vi "Mod_OFDM_Config_Data_Source.vi"(0 "Configuration in":variant=variant("Attribute Names"=variant(cluster{"Data Source Pool":string, "Modulator Source Pool":string, "OFDM SYMBOL POOL":string, "Symbol Table":string, "Sub Carrier Selection":string, "OFDM Frame":string, "FRAME Table":string, "Pulse Shaping":string} {"Data Source Pool"="Data Source ", "Modulator Source Pool"="Modulator Source Pool ", "OFDM SYMBOL POOL"="OFDM SYMBOL POOL", "Symbol Table"="Symbol Table", "Sub Carrier Selection"="Sub Carrier Selection", "OFDM Frame"="OFDM Frame", "FRAME Table"="FRAME Table", "Pulse Shaping"="Pulse Shaping"}), "Data Source "=variant(cluster{"mode (PN)":enum16{"PN", "pattern", "user"}, "PN sequence order (9)":i32, "Invert Output Bits":enum16{"No", "Yes"}, "Register Initial State":u32, "User base bit pattern":i8[], "base bit pattern (00001111)":enum16{"0", "1", "01", "0011", "00001111"}, "Reset to Initial State":enum16{"Every OFDM Frame", "Every OFDM Symbol", "Every Sub Carrier"}}[] [{"mode (PN)"=enum."PN", "PN sequence order (9)"=9, "Invert Output Bits"=enum."No", "Register Initial State"=3602873842, "User base bit pattern"=[], "base bit pattern (00001111)"=enum."00001111", "Reset to Initial State"=enum."Every OFDM Frame"}, {"mode (PN)"=enum."PN", "PN sequence order (9)"=9, "Invert Output Bits"=enum."No", "Register Initial State"=3602873842, "User base bit pattern"=[], "base bit pattern (00001111)"=enum."00001111", "Reset to Initial State"=enum."Every OFDM Frame"}, {"mode (PN)"=enum."PN", "PN sequence order (9)"=9, "Invert Output Bits"=enum."No", "Register Initial State"=3602873842, "User base bit pattern"=[], "base bit pattern (00001111)"=enum."00001111", "Reset to Initial State"=enum."Every OFDM Frame"}, {"mode (PN)"=enum."PN", "PN sequence order (9)"=9, "Invert Output Bits"=enum."No", "Register Initial State"=3602873842, "User base bit pattern"=[], "base bit pattern (00001111)"=enum."00001111", "Reset to Initial State"=enum."Every OFDM Frame"}]), "FRAME Table"=variant(string[][] [["No_Name", "  1", "  1"], ["No_Name", "  1", "  2"]]), "Modulator Source Pool "=variant(cluster{"M-QAM":enum16{"4", "16", "64", "256"}, "M-PSK":enum16{"2", "4", "8", "16", "32", "64", "128", "256"}, "Type of Modulation":enum16{"PSK", "QAM"}, "PSK":cluster{"differential PSK":enum16{"disable", "enable"}, "PSK type":enum16{"normal", "shifted", "offset"}}}[] [{"M-QAM"=enum."4", "M-PSK"=enum."2", "Type of Modulation"=enum."PSK", "PSK"={"differential PSK"=enum."disable", "PSK type"=enum."normal"}}, {"M-QAM"=enum."4", "M-PSK"=enum."2", "Type of Modulation"=enum."PSK", "PSK"={"differential PSK"=enum."disable", "PSK type"=enum."normal"}}, {"M-QAM"=enum."4", "M-PSK"=enum."2", "Type of Modulation"=enum."PSK", "PSK"={"differential PSK"=enum."disable", "PSK type"=enum."normal"}}, {"M-QAM"=enum."4", "M-PSK"=enum."2", "Type of Modulation"=enum."PSK", "PSK"={"differential PSK"=enum."disable", "PSK type"=enum."normal"}}]), "No_Name"=variant(cluster{"Sub Carrier Selection":cluster{"Sub Carrier":bool, "Data Source":u16, "Modulator":u16}[], "OFDM Parameters":cluster{"# of Sub Carrier":i32, "Length Of Cylic Prefix":i32}} {"Sub Carrier Selection"=[{"Sub Carrier"=TRUE, "Data Source"=0, "Modulator"=0}, {"Sub Carrier"=TRUE, "Data Source"=0, "Modulator"=0}, {"Sub Carrier"=TRUE, "Data Source"=0, "Modulator"=0}, {"Sub Carrier"=TRUE, "Data Source"=0, "Modulator"=0}, {"Sub Carrier"=TRUE, "Data Source"=0, "Modulator"=0}, {"Sub Carrier"=TRUE, "Data Source"=0, "Modulator"=0}, {"Sub Carrier"=TRUE, "Data Source"=0, "Modulator"=0}, {"Sub Carrier"=TRUE, "Data Source"=0, "Modulator"=0}, {"Sub Carrier"=TRUE, "Data Source"=0, "Modulator"=0}, {"Sub Carrier"=TRUE, "Data Source"=0, "Modulator"=0}, {"Sub Carrier"=TRUE, "Data Source"=0, "Modulator"=0}, {"Sub Carrier"=TRUE, "Data Source"=0, "Modulator"=0}, {"Sub Carrier"=TRUE, "Data Source"=0, "Modulator"=0}, {"Sub Carrier"=TRUE, "Data Source"=0, "Modulator"=0}, {"Sub Carrier"=TRUE, "Data Source"=0, "Modulator"=0}, {"Sub Carrier"=TRUE, "Data Source"=0, "Modulator"=0}, {"Sub Carrier"=TRUE, "Data Source"=0, "Modulator"=0}, {"Sub Carrier"=TRUE, "Data Source"=0, "Modulator"=0}, {"Sub Carrier"=TRUE, "Data Source"=0, "Modulator"=0}, {"Sub Carrier"=TRUE, "Data Source"=0, "Modulator"=0}, {"Sub Carrier"=TRUE, "Data Source"=0, "Modulator"=0}, {"Sub Carrier"=TRUE, "Data Source"=0, "Modulator"=0}, {"Sub Carrier"=TRUE, "Data Source"=0, "Modulator"=0}, {"Sub Carrier"=TRUE, "Data Source"=0, "Modulator"=0}, {"Sub Carrier"=TRUE, "Data Source"=0, "Modulator"=0}, {"Sub Carrier"=TRUE, "Data Source"=0, "Modulator"=0}, {"Sub Carrier"=TRUE, "Data Source"=0, "Modulator"=0}, {"Sub Carrier"=TRUE, "Data Source"=0, "Modulator"=0}, {"Sub Carrier"=TRUE, "Data Source"=0, "Modulator"=0}, {"Sub Carrier"=TRUE, "Data Source"=0, "Modulator"=0}, {"Sub Carrier"=TRUE, "Data Source"=0, "Modulator"=0}, {"Sub Carrier"=TRUE, "Data Source"=0, "Modulator"=0}, {"Sub Carrier"=TRUE, "Data Source"=0, "Modulator"=0}, {"Sub Carrier"=TRUE, "Data Source"=0, "Modulator"=0}, {"Sub Carrier"=TRUE, "Data Source"=0, "Modulator"=0}, {"Sub Carrier"=TRUE, "Data Source"=0, "Modulator"=0}, {"Sub Carrier"=TRUE, "Data Source"=0, "Modulator"=0}, {"Sub Carrier"=TRUE, "Data Source"=0, "Modulator"=0}, {"Sub Carrier"=TRUE, "Data Source"=0, "Modulator"=0}, {"Sub Carrier"=TRUE, "Data Source"=0, "Modulator"=0}, {"Sub Carrier"=TRUE, "Data Source"=0, "Modulator"=0}, {"Sub Carrier"=TRUE, "Data Source"=0, "Modulator"=0}, {"Sub Carrier"=TRUE, "Data Source"=0, "Modulator"=0}, {"Sub Carrier"=TRUE, "Data Source"=0, "Modulator"=0}, {"Sub Carrier"=TRUE, "Data Source"=0, "Modulator"=0}, {"Sub Carrier"=TRUE, "Data Source"=0, "Modulator"=0}, {"Sub Carrier"=TRUE, "Data Source"=0, "Modulator"=0}, {"Sub Carrier"=TRUE, "Data Source"=0, "Modulator"=0}, {"Sub Carrier"=TRUE, "Data Source"=0, "Modulator"=0}, {"Sub Carrier"=TRUE, "Data Source"=0, "Modulator"=0}, {"Sub Carrier"=TRUE, "Data Source"=0, "Modulator"=0}, {"Sub Carrier"=TRUE, "Data Source"=0, "Modulator"=0}, {"Sub Carrier"=TRUE, "Data Source"=0, "Modulator"=0}, {"Sub Carrier"=TRUE, "Data Source"=0, "Modulator"=0}, {"Sub Carrier"=TRUE, "Data Source"=0, "Modulator"=0}, {"Sub Carrier"=TRUE, "Data Source"=0, "Modulator"=0}, {"Sub Carrier"=TRUE, "Data Source"=0, "Modulator"=0}, {"Sub Carrier"=TRUE, "Data Source"=0, "Modulator"=0}, {"Sub Carrier"=TRUE, "Data Source"=0, "Modulator"=0}, {"Sub Carrier"=TRUE, "Data Source"=0, "Modulator"=0}, {"Sub Carrier"=TRUE, "Data Source"=0, "Modulator"=0}, {"Sub Carrier"=TRUE, "Data Source"=0, "Modulator"=0}, {"Sub Carrier"=TRUE, "Data Source"=0, "Modulator"=0}, {"Sub Carrier"=TRUE, "Data Source"=0, "Modulator"=0}], "OFDM Parameters"={"# of Sub Carrier"=64, "Length Of Cylic Prefix"=16}}), "OFDM Frame"=variant(cluster{"Symbol Name":string, "# of Symbols":i32}[] [{"Symbol Name"="No_Name", "# of Symbols"=1}, {"Symbol Name"="No_Name", "# of Symbols"=1}]), "OFDM SYMBOL POOL"=variant(string[] ["No_Name"]), "Pulse Shaping"=variant(cluster{"System Filter":cluster{"TX Filter":enum16{"none", "Raised Cosine", "Root Raised Cos"}, "Alpha":dbl, "filter length":i32}, "Modulation system parameters":cluster{"samples per symbol (16)":u32}, "symbol rate (Hz)":dbl} {"System Filter"={"TX Filter"=enum."Root Raised Cos", "Alpha"=0.5, "filter length"=8}, "Modulation system parameters"={"samples per symbol (16)"=16}, "symbol rate (Hz)"=100000.0}), "Sub Carrier Selection"=variant(cluster{"Sub Carrier Selection":cluster{"Sub Carrier":bool, "Data Source":u16, "Modulator":u16}[], "OFDM Parameters":cluster{"# of Sub Carrier":i32, "Length Of Cylic Prefix":i32}} {"Sub Carrier Selection"=array[10000 elements], "OFDM Parameters"={"# of Sub Carrier"=64, "Length Of Cylic Prefix"=16}}), "Symbol Table"=variant(string[][] [["-32", " ON", "0", "0"], ["-31", " ON", "0", "0"], ["-30", " ON", "0", "0"], ["-29", " ON", "0", "0"], ["-28", " ON", "0", "0"], ["-27", " ON", "0", "0"], ["-26", " ON", "0", "0"], ["-25", " ON", "0", "0"], ["-24", " ON", "0", "0"], ["-23", " ON", "0", "0"], ["-22", " ON", "0", "0"], ["-21", " ON", "0", "0"], ["-20", " ON", "0", "0"], ["-19", " ON", "0", "0"], ["-18", " ON", "0", "0"], ["-17", " ON", "0", "0"], ["-16", " ON", "0", "0"], ["-15", " ON", "0", "0"], ["-14", " ON", "0", "0"], ["-13", " ON", "0", "0"], ["-12", " ON", "0", "0"], ["-11", " ON", "0", "0"], ["-10", " ON", "0", "0"], ["-9", " ON", "0", "0"], ["-8", " ON", "0", "0"], ["-7", " ON", "0", "0"], ["-6", " ON", "0", "0"], ["-5", " ON", "0", "0"], ["-4", " ON", "0", "0"], ["-3", " ON", "0", "0"], ["-2", " ON", "0", "0"], ["-1", " ON", "0", "0"], ["0", " ON", "0", "0"], ["+1", " ON", "0", "0"], ["+2", " ON", "0", "0"], ["+3", " ON", "0", "0"], ["+4", " ON", "0", "0"], ["+5", " ON", "0", "0"], ["+6", " ON", "0", "0"], ["+7", " ON", "0", "0"], ["+8", " ON", "0", "0"], ["+9", " ON", "0", "0"], ["+10", " ON", "0", "0"], ["+11", " ON", "0", "0"], ["+12", " ON", "0", "0"], ["+13", " ON", "0", "0"], ["+14", " ON", "0", "0"], ["+15", " ON", "0", "0"], ["+16", " ON", "0", "0"], ["+17", " ON", "0", "0"], ["+18", " ON", "0", "0"], ["+19", " ON", "0", "0"], ["+20", " ON", "0", "0"], ["+21", " ON", "0", "0"], ["+22", " ON", "0", "0"], ["+23", " ON", "0", "0"], ["+24", " ON", "0", "0"], ["+25", " ON", "0", "0"], ["+26", " ON", "0", "0"], ["+27", " ON", "0", "0"], ["+28", " ON", "0", "0"], ["+29", " ON", "0", "0"], ["+30", " ON", "0", "0"], ["+31", " ON", "0", "0"]])), 7 "Pool of Data Sources":T1=[{"mode (PN)"=enum."PN", "PN sequence order (9)"=9, "Invert Output Bits"=enum."No", "Register Initial State "=3602873842, "User base bit pattern"=[], "base bit pattern (00001111)"=enum."00001111", "Reset to Initial State"=enum."Every OFDM Frame"}, {"mode (PN)"=enum."PN", "PN sequence order (9)"=9, "Invert Output Bits"=enum."No", "Register Initial State "=3602873842, "User base bit pattern"=[], "base bit pattern (00001111)"=enum."00001111", "Reset to Initial State"=enum."Every OFDM Frame"}, {"mode (PN)"=enum."PN", "PN sequence order (9)"=9, "Invert Output Bits"=enum."No", "Register Initial State "=3602873842, "User base bit pattern"=[], "base bit pattern (00001111)"=enum."00001111", "Reset to Initial State"=enum."Every OFDM Frame"}, {"mode (PN)"=enum."PN", "PN sequence order (9)"=9, "Invert Output Bits"=enum."No", "Register Initial State "=3602873842, "User base bit pattern"=[], "base bit pattern (00001111)"=enum."00001111", "Reset to Initial State"=enum."Every OFDM Frame"}] {"Register Initial State" format="%08x"}, 11 "error in":errorcluster) -> (4 "Configuration out":variant=variant("Attribute Names"=variant(cluster{"Data Source Pool":string, "Modulator Source Pool":string, "OFDM SYMBOL POOL":string, "Symbol Table":string, "Sub Carrier Selection":string, "OFDM Frame":string, "FRAME Table":string, "Pulse Shaping":string} {"Data Source Pool"="Data Source ", "Modulator Source Pool"="Modulator Source Pool ", "OFDM SYMBOL POOL"="OFDM SYMBOL POOL", "Symbol Table"="Symbol Table", "Sub Carrier Selection"="Sub Carrier Selection", "OFDM Frame"="OFDM Frame", "FRAME Table"="FRAME Table", "Pulse Shaping"="Pulse Shaping"}), "Data Source "=variant(cluster{"mode (PN)":enum16{"PN", "pattern", "user"}, "PN sequence order (9)":i32, "Invert Output Bits":enum16{"No", "Yes"}, "Register Initial State":u32, "User base bit pattern":i8[], "base bit pattern (00001111)":enum16{"0", "1", "01", "0011", "00001111"}, "Reset to Initial State":enum16{"Every OFDM Frame", "Every OFDM Symbol", "Every Sub Carrier"}}[] [{"mode (PN)"=enum."PN", "PN sequence order (9)"=9, "Invert Output Bits"=enum."No", "Register Initial State"=3602873842, "User base bit pattern"=[], "base bit pattern (00001111)"=enum."00001111", "Reset to Initial State"=enum."Every OFDM Frame"}, {"mode (PN)"=enum."PN", "PN sequence order (9)"=9, "Invert Output Bits"=enum."No", "Register Initial State"=3602873842, "User base bit pattern"=[], "base bit pattern (00001111)"=enum."00001111", "Reset to Initial State"=enum."Every OFDM Frame"}, {"mode (PN)"=enum."PN", "PN sequence order (9)"=9, "Invert Output Bits"=enum."No", "Register Initial State"=3602873842, "User base bit pattern"=[], "base bit pattern (00001111)"=enum."00001111", "Reset to Initial State"=enum."Every OFDM Frame"}, {"mode (PN)"=enum."PN", "PN sequence order (9)"=9, "Invert Output Bits"=enum."No", "Register Initial State"=3602873842, "User base bit pattern"=[], "base bit pattern (00001111)"=enum."00001111", "Reset to Initial State"=enum."Every OFDM Frame"}]), "FRAME Table"=variant(string[][] [["No_Name", "  1", "  1"], ["No_Name", "  1", "  2"]]), "Modulator Source Pool "=variant(cluster{"M-QAM":enum16{"4", "16", "64", "256"}, "M-PSK":enum16{"2", "4", "8", "16", "32", "64", "128", "256"}, "Type of Modulation":enum16{"PSK", "QAM"}, "PSK":cluster{"differential PSK":enum16{"disable", "enable"}, "PSK type":enum16{"normal", "shifted", "offset"}}}[] [{"M-QAM"=enum."4", "M-PSK"=enum."2", "Type of Modulation"=enum."PSK", "PSK"={"differential PSK"=enum."disable", "PSK type"=enum."normal"}}, {"M-QAM"=enum."4", "M-PSK"=enum."2", "Type of Modulation"=enum."PSK", "PSK"={"differential PSK"=enum."disable", "PSK type"=enum."normal"}}, {"M-QAM"=enum."4", "M-PSK"=enum."2", "Type of Modulation"=enum."PSK", "PSK"={"differential PSK"=enum."disable", "PSK type"=enum."normal"}}, {"M-QAM"=enum."4", "M-PSK"=enum."2", "Type of Modulation"=enum."PSK", "PSK"={"differential PSK"=enum."disable", "PSK type"=enum."normal"}}]), "No_Name"=variant(cluster{"Sub Carrier Selection":cluster{"Sub Carrier":bool, "Data Source":u16, "Modulator":u16}[], "OFDM Parameters":cluster{"# of Sub Carrier":i32, "Length Of Cylic Prefix":i32}} {"Sub Carrier Selection"=[{"Sub Carrier"=TRUE, "Data Source"=0, "Modulator"=0}, {"Sub Carrier"=TRUE, "Data Source"=0, "Modulator"=0}, {"Sub Carrier"=TRUE, "Data Source"=0, "Modulator"=0}, {"Sub Carrier"=TRUE, "Data Source"=0, "Modulator"=0}, {"Sub Carrier"=TRUE, "Data Source"=0, "Modulator"=0}, {"Sub Carrier"=TRUE, "Data Source"=0, "Modulator"=0}, {"Sub Carrier"=TRUE, "Data Source"=0, "Modulator"=0}, {"Sub Carrier"=TRUE, "Data Source"=0, "Modulator"=0}, {"Sub Carrier"=TRUE, "Data Source"=0, "Modulator"=0}, {"Sub Carrier"=TRUE, "Data Source"=0, "Modulator"=0}, {"Sub Carrier"=TRUE, "Data Source"=0, "Modulator"=0}, {"Sub Carrier"=TRUE, "Data Source"=0, "Modulator"=0}, {"Sub Carrier"=TRUE, "Data Source"=0, "Modulator"=0}, {"Sub Carrier"=TRUE, "Data Source"=0, "Modulator"=0}, {"Sub Carrier"=TRUE, "Data Source"=0, "Modulator"=0}, {"Sub Carrier"=TRUE, "Data Source"=0, "Modulator"=0}, {"Sub Carrier"=TRUE, "Data Source"=0, "Modulator"=0}, {"Sub Carrier"=TRUE, "Data Source"=0, "Modulator"=0}, {"Sub Carrier"=TRUE, "Data Source"=0, "Modulator"=0}, {"Sub Carrier"=TRUE, "Data Source"=0, "Modulator"=0}, {"Sub Carrier"=TRUE, "Data Source"=0, "Modulator"=0}, {"Sub Carrier"=TRUE, "Data Source"=0, "Modulator"=0}, {"Sub Carrier"=TRUE, "Data Source"=0, "Modulator"=0}, {"Sub Carrier"=TRUE, "Data Source"=0, "Modulator"=0}, {"Sub Carrier"=TRUE, "Data Source"=0, "Modulator"=0}, {"Sub Carrier"=TRUE, "Data Source"=0, "Modulator"=0}, {"Sub Carrier"=TRUE, "Data Source"=0, "Modulator"=0}, {"Sub Carrier"=TRUE, "Data Source"=0, "Modulator"=0}, {"Sub Carrier"=TRUE, "Data Source"=0, "Modulator"=0}, {"Sub Carrier"=TRUE, "Data Source"=0, "Modulator"=0}, {"Sub Carrier"=TRUE, "Data Source"=0, "Modulator"=0}, {"Sub Carrier"=TRUE, "Data Source"=0, "Modulator"=0}, {"Sub Carrier"=TRUE, "Data Source"=0, "Modulator"=0}, {"Sub Carrier"=TRUE, "Data Source"=0, "Modulator"=0}, {"Sub Carrier"=TRUE, "Data Source"=0, "Modulator"=0}, {"Sub Carrier"=TRUE, "Data Source"=0, "Modulator"=0}, {"Sub Carrier"=TRUE, "Data Source"=0, "Modulator"=0}, {"Sub Carrier"=TRUE, "Data Source"=0, "Modulator"=0}, {"Sub Carrier"=TRUE, "Data Source"=0, "Modulator"=0}, {"Sub Carrier"=TRUE, "Data Source"=0, "Modulator"=0}, {"Sub Carrier"=TRUE, "Data Source"=0, "Modulator"=0}, {"Sub Carrier"=TRUE, "Data Source"=0, "Modulator"=0}, {"Sub Carrier"=TRUE, "Data Source"=0, "Modulator"=0}, {"Sub Carrier"=TRUE, "Data Source"=0, "Modulator"=0}, {"Sub Carrier"=TRUE, "Data Source"=0, "Modulator"=0}, {"Sub Carrier"=TRUE, "Data Source"=0, "Modulator"=0}, {"Sub Carrier"=TRUE, "Data Source"=0, "Modulator"=0}, {"Sub Carrier"=TRUE, "Data Source"=0, "Modulator"=0}, {"Sub Carrier"=TRUE, "Data Source"=0, "Modulator"=0}, {"Sub Carrier"=TRUE, "Data Source"=0, "Modulator"=0}, {"Sub Carrier"=TRUE, "Data Source"=0, "Modulator"=0}, {"Sub Carrier"=TRUE, "Data Source"=0, "Modulator"=0}, {"Sub Carrier"=TRUE, "Data Source"=0, "Modulator"=0}, {"Sub Carrier"=TRUE, "Data Source"=0, "Modulator"=0}, {"Sub Carrier"=TRUE, "Data Source"=0, "Modulator"=0}, {"Sub Carrier"=TRUE, "Data Source"=0, "Modulator"=0}, {"Sub Carrier"=TRUE, "Data Source"=0, "Modulator"=0}, {"Sub Carrier"=TRUE, "Data Source"=0, "Modulator"=0}, {"Sub Carrier"=TRUE, "Data Source"=0, "Modulator"=0}, {"Sub Carrier"=TRUE, "Data Source"=0, "Modulator"=0}, {"Sub Carrier"=TRUE, "Data Source"=0, "Modulator"=0}, {"Sub Carrier"=TRUE, "Data Source"=0, "Modulator"=0}, {"Sub Carrier"=TRUE, "Data Source"=0, "Modulator"=0}, {"Sub Carrier"=TRUE, "Data Source"=0, "Modulator"=0}], "OFDM Parameters"={"# of Sub Carrier"=64, "Length Of Cylic Prefix"=16}}), "OFDM Frame"=variant(cluster{"Symbol Name":string, "# of Symbols":i32}[] [{"Symbol Name"="No_Name", "# of Symbols"=1}, {"Symbol Name"="No_Name", "# of Symbols"=1}]), "OFDM SYMBOL POOL"=variant(string[] ["No_Name"]), "Pulse Shaping"=variant(cluster{"System Filter":cluster{"TX Filter":enum16{"none", "Raised Cosine", "Root Raised Cos"}, "Alpha":dbl, "filter length":i32}, "Modulation system parameters":cluster{"samples per symbol (16)":u32}, "symbol rate (Hz)":dbl} {"System Filter"={"TX Filter"=enum."Root Raised Cos", "Alpha"=0.5, "filter length"=8}, "Modulation system parameters"={"samples per symbol (16)"=16}, "symbol rate (Hz)"=100000.0}), "Sub Carrier Selection"=variant(cluster{"Sub Carrier Selection":cluster{"Sub Carrier":bool, "Data Source":u16, "Modulator":u16}[], "OFDM Parameters":cluster{"# of Sub Carrier":i32, "Length Of Cylic Prefix":i32}} {"Sub Carrier Selection"=array[10000 elements], "OFDM Parameters"={"# of Sub Carrier"=64, "Length Of Cylic Prefix"=16}}), "Symbol Table"=variant(string[][] [["-32", " ON", "0", "0"], ["-31", " ON", "0", "0"], ["-30", " ON", "0", "0"], ["-29", " ON", "0", "0"], ["-28", " ON", "0", "0"], ["-27", " ON", "0", "0"], ["-26", " ON", "0", "0"], ["-25", " ON", "0", "0"], ["-24", " ON", "0", "0"], ["-23", " ON", "0", "0"], ["-22", " ON", "0", "0"], ["-21", " ON", "0", "0"], ["-20", " ON", "0", "0"], ["-19", " ON", "0", "0"], ["-18", " ON", "0", "0"], ["-17", " ON", "0", "0"], ["-16", " ON", "0", "0"], ["-15", " ON", "0", "0"], ["-14", " ON", "0", "0"], ["-13", " ON", "0", "0"], ["-12", " ON", "0", "0"], ["-11", " ON", "0", "0"], ["-10", " ON", "0", "0"], ["-9", " ON", "0", "0"], ["-8", " ON", "0", "0"], ["-7", " ON", "0", "0"], ["-6", " ON", "0", "0"], ["-5", " ON", "0", "0"], ["-4", " ON", "0", "0"], ["-3", " ON", "0", "0"], ["-2", " ON", "0", "0"], ["-1", " ON", "0", "0"], ["0", " ON", "0", "0"], ["+1", " ON", "0", "0"], ["+2", " ON", "0", "0"], ["+3", " ON", "0", "0"], ["+4", " ON", "0", "0"], ["+5", " ON", "0", "0"], ["+6", " ON", "0", "0"], ["+7", " ON", "0", "0"], ["+8", " ON", "0", "0"], ["+9", " ON", "0", "0"], ["+10", " ON", "0", "0"], ["+11", " ON", "0", "0"], ["+12", " ON", "0", "0"], ["+13", " ON", "0", "0"], ["+14", " ON", "0", "0"], ["+15", " ON", "0", "0"], ["+16", " ON", "0", "0"], ["+17", " ON", "0", "0"], ["+18", " ON", "0", "0"], ["+19", " ON", "0", "0"], ["+20", " ON", "0", "0"], ["+21", " ON", "0", "0"], ["+22", " ON", "0", "0"], ["+23", " ON", "0", "0"], ["+24", " ON", "0", "0"], ["+25", " ON", "0", "0"], ["+26", " ON", "0", "0"], ["+27", " ON", "0", "0"], ["+28", " ON", "0", "0"], ["+29", " ON", "0", "0"], ["+30", " ON", "0", "0"], ["+31", " ON", "0", "0"]])), 8 "Pool of Data Sources":T1=[{"mode (PN)"=enum."PN", "PN sequence order (9)"=9, "Invert Output Bits"=enum."No", "Register Initial State "=3602873842, "User base bit pattern"=[], "base bit pattern (00001111)"=enum."00001111", "Reset to Initial State"=enum."Every OFDM Frame"}, {"mode (PN)"=enum."PN", "PN sequence order (9)"=9, "Invert Output Bits"=enum."No", "Register Initial State "=3602873842, "User base bit pattern"=[], "base bit pattern (00001111)"=enum."00001111", "Reset to Initial State"=enum."Every OFDM Frame"}, {"mode (PN)"=enum."PN", "PN sequence order (9)"=9, "Invert Output Bits"=enum."No", "Register Initial State "=3602873842, "User base bit pattern"=[], "base bit pattern (00001111)"=enum."00001111", "Reset to Initial State"=enum."Every OFDM Frame"}, {"mode (PN)"=enum."PN", "PN sequence order (9)"=9, "Invert Output Bits"=enum."No", "Register Initial State "=3602873842, "User base bit pattern"=[], "base bit pattern (00001111)"=enum."00001111", "Reset to Initial State"=enum."Every OFDM Frame"}] {"Register Initial State" format="%08x"}, 15 "error out":errorcluster)   [LabVIEW 2010]
uses:
  Controls(Type_DEf)/Pool of Data Source Control.ctl
panel:
  in  "Cancel Operation":bool
  in  "Apply Settings":bool
  # "* Initializes the PN Generator\n\nevery Sub Carrier:\nreset for each sub carrier\n\nevery OFDM Symb:\nreset at the beginning of every OFDM symbol\n\nevery Frame:\nreset at the beginning of every frame"
  # "*"
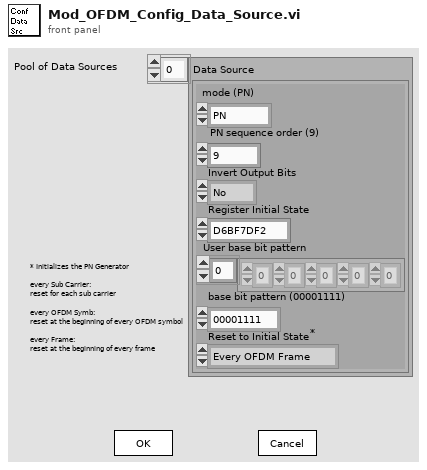
[diagram p1: front panel]
types:
  T1 = typedef "Pool of Data Source Control.ctl" = cluster{"mode (PN)":enum16{"PN", "pattern", "user"}, "PN sequence order (9)":i32, "Invert Output Bits":enum16{"No", "Yes"}, "Register Initial State ":u32, "User base bit pattern":i8[], "base bit pattern (00001111)":enum16{"0", "1", "01", "0011", "00001111"}, "Reset to Initial State":enum16{"Every OFDM Frame", "Every OFDM Symbol", "Every Sub Carrier"}}[]
  T2 = cluster{"mode (PN)":enum16{"PN", "pattern", "user"}, "PN sequence order (9)":i32, "Invert Output Bits":enum16{"No", "Yes"}, "Register Initial State ":u32, "User base bit pattern":i8[], "base bit pattern (00001111)":enum16{"0", "1", "01", "0011", "00001111"}, "Reset to Initial State":enum16{"Every OFDM Frame", "Every OFDM Symbol", "Every Sub Carrier"}}[]
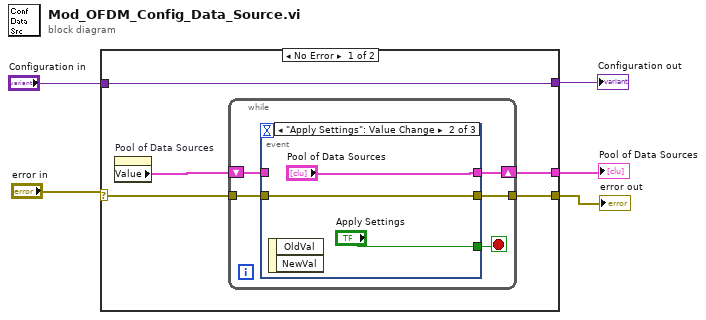
[diagram p0: block diagram]
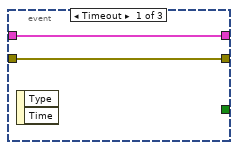
[diagram p2: hidden frame]
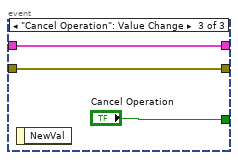
[diagram p3: hidden frame]
diagram:
  n1 = case shown="No Error" "error in" {
    selector: "error in" -> [w9 w24]
    tunnel: [w10 _] -> w1
    tunnel: [w8 w24] -> w4
    tunnel: "Configuration in" -> [w7 _]
    tunnel: [w7 _] -> w2
    frame No Error {
      n2 = property on="Pool of Data Sources" class="Arr (strict)"() -> ("Value"=w6:T2)  [unwired: 2 in, 2 out]
      n3 = while {
        shift-right: [w14] -> w10
        shift-left: w6 -> [w13]
        tunnel: w9 -> [w11]
        tunnel: [w12] -> w8
        stop <- w15 stop-if-true
        n4 = event shown="[1] \"Apply Settings\": Value Change" {
          selector: _ -> [_ _ _]
          dyn-events: _ -> [_ _ _]
          timeout: _ -> [_ _ _]
          tunnel: [_ "Apply Settings" "Cancel Operation"] -> w15
          tunnel: [w17 "Pool of Data Sources" w21] -> w14
          tunnel: w13 -> [w17 _ w21]
          tunnel: [w16 w19 w22] -> w12
          tunnel: w11 -> [w16 w19 w22]
          event Timeout {
            n5 = event-data() -> ()  [unwired: 1 in, 2 out]
          }
          event "Apply Settings": Value Change {
            n6 = event-data() -> ()  [unwired: 1 in, 2 out]
          }
          event "Cancel Operation": Value Change {
            n7 = event-data() -> ()  [unwired: 1 in, 1 out]
          }
        }
      }
    }
    frame Error {
    }
  }
  "Pool of Data Sources" <- w1
  "error out" <- w4
  "Configuration out" <- w2
